vi "Read modulationConfig.vi"(8 "error in (no error)":errorcluster, 11 "BuckBoost configuration in":refnum<class "BuckBoost configuration.lvclass">) -> (0 "error out":errorcluster, 2 "modulationConfig":T1 {"modulationRate" format="%#_6p"; "Deadband" format="%#_6p"; "SwitchingSpeed" format="%#_6p"}, 3 "BuckBoost configuration out":refnum<class "BuckBoost configuration.lvclass">)   [LabVIEW 2017, in "BuckBoost configuration.lvclass"]
uses:
  BuckBoost configuration.lvclass
  <vilib>/NI/PowerElectronicsControl/Buck-Boost/RealTime/modulationConfig.ctl
  BuckBoost configuration.lvclass/BuckBoost configuration.ctl
  <vilib>/NI/PowerElectronicsControl/Buck-Boost/RealTime/BuckBoostInterface.lvlib
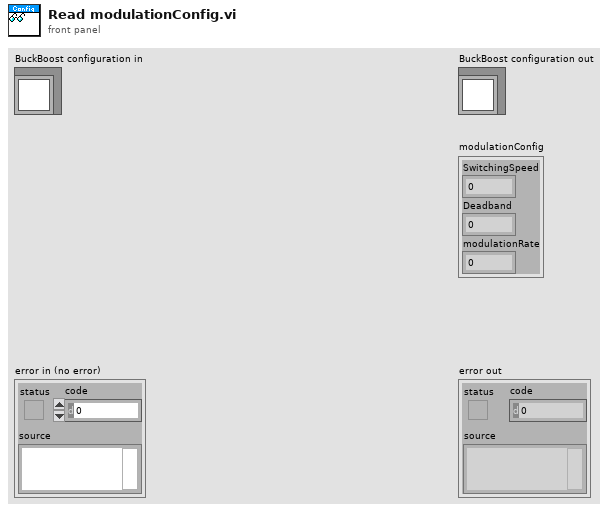
[diagram p1: front panel]
types:
  T1 = typedef "BuckBoostInterface.lvlib/modulationConfig.ctl" = cluster{"SwitchingSpeed":dbl, "Deadband":dbl, "modulationRate":dbl}
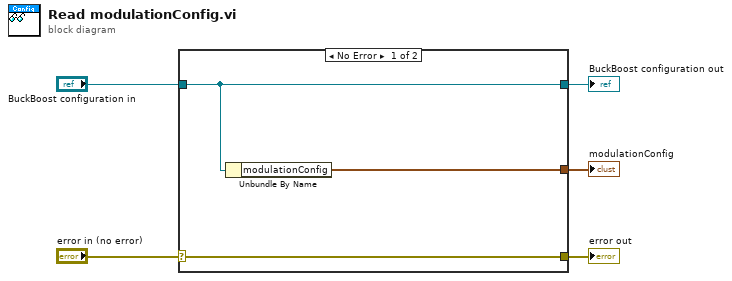
[diagram p0: block diagram]
diagram:
  n1 = case shown="No Error" "error in (no error)" {
    selector: "error in (no error)" -> [w8 w9]
    tunnel: [w8 w9] -> w4
    tunnel: [w7 w10] -> w2
    tunnel: "BuckBoost configuration in" -> [w7 w10]
    tunnel: [w6 _] -> w1
    frame No Error {
      n2 = Unbundle By Name(w7) -> ("modulationConfig"=w6:T1)
    }
    frame Error {
    }
  }
  "error out" <- w4
  "BuckBoost configuration out" <- w2
  "modulationConfig" <- w1
